vi "Test NES.vi"() -> ()   [LabVIEW 2019]
uses:
  src/Instrument.DAQ/Typedefs/Get State-enum.ctl
  src/Instrument UI.Lockin/Typedefs/UI.Configuration--Cluster.ctl
  src/Instrument.DAQ/Typedefs/Configuration.Channels--Cluster.ctl
  src/Instrument.DAQ/Typedefs/AO.Channel--Cluster--Array.ctl
  src/Instrument.DAQ/Typedefs/AO.Channel--Cluster.ctl
  src/Instrument.DAQ/Typedefs/AO.Channel.Function--Enum.ctl
  src/Instrument.DAQ/Typedefs/AI.Channel--Cluster--Array.ctl
  src/Instrument.DAQ/Typedefs/AI.Channel--Cluster.ctl
  src/Instrument.DAQ/Typedefs/REF.Channel--Cluster--Array.ctl
  src/Instrument.DAQ/Typedefs/REF.Channel--Cluster.ctl
  src/Instrument.DAQ/Typedefs/DAQ.Configuration--Cluster--Array.ctl
  src/Instrument.DAQ/Typedefs/DAQ.Configuration--Cluster.ctl
  src/Instrument.DAQ/Typedefs/DAQ.Config.AO.Range--enum.ctl
  src/Instrument.DAQ/Typedefs/DAQ.Config.AI.Range--enum.ctl
  src/Instrument.DAQ/Typedefs/DAQ.Config.AI.Coupling--enum.ctl
  src/Instrument.DAQ/Typedefs/DAQ.TerminalConfiguration--ring.ctl
  src/Instrument.DAQ/Typedefs/DAQ.Sampling--Cluster.ctl
  src/Instrument.DAQ/Typedefs/DAQ.Sampling.Sampling--Cluster.ctl
  src/Instrument.DAQ/Typedefs/DAQ.Sampling.Fs Mode--enum.ctl
  src/Instrument.DAQ/Typedefs/DAQ.Calibration--Cluster--Array.ctl
  src/Instrument.DAQ/Typedefs/DAQ.Calibration--Cluster.ctl
  src/Instrument.DAQ/Typedefs/Simulation Mode--enum.ctl
  src/Instrument.DAQ/Typedefs/Configuration.Prefilter--Cluster.ctl
  src/Instrument.DAQ/Typedefs/Channel.GainsAndOffsets--Cluster.ctl
  src/Instrument.DAQ/Typedefs/Channel.Gain--Cluster--Array.ctl
  src/Instrument.DAQ/Typedefs/Channel.Gain--Cluster.ctl
  src/Instrument.DAQ/Typedefs/Configuration.AmplitudeLimit--Cluster.ctl
  src/Instrument.DAQ/Typedefs/Configuration.DCLimit--Cluster.ctl
  src/Instrument.DAQ/Typedefs/Configuration.LinkFrequencies--Cluster.ctl
  src/Instrument.DAQ/Typedefs/Sweep.Configuration--Cluster.ctl
  src/Instrument.DAQ/Typedefs/Sweep.Channel--Cluster--Array.ctl
  src/Instrument.DAQ/Typedefs/Sweep.Channel--Cluster.ctl
  src/Instrument.DAQ/Typedefs/Sweep.Pattern--Enum.ctl
  src/Instrument UI.Lockin/Typedefs/Display-Enum.ctl
  src/Instrument.DAQ/Typedefs/Configuration.DutyCycle--Cluster.ctl
  src/Instrument UI.Lockin/Typedefs/UI.References--Cluster.ctl
  src/Instrument UI.Lockin/Typedefs/UI.References.Booleans--Cluster.ctl
  src/Instrument UI.Lockin/Typedefs/UI.References.Clusters--Cluster.ctl
  src/Instrument UI.Lockin/Typedefs/UI.References.Graphs--Cluster.ctl
  src/Instrument.Lockin/Typedefs/Lockin.getAllData--Cluster.ctl
  src/Instrument.DAQ/Typedefs/PublicEvents--DAQ.getWaveforms.ctl
  src/Instrument.DAQ/Typedefs/Results--Cluster.ctl
  src/Instrument.DAQ/Typedefs/PublicEvents--DAQ.getSweepWaveforms.ctl
  <userlib>/LevyLab/Configuration/Configuration.lvclass
  src/Instrument.DAQ/Instrument.DAQ.lvclass
  src/Instrument.Lockin/Instrument.Lockin.lvclass
  src/Instrument UI.Lockin/Instrument UI.Lockin.lvclass
  <vilib>/measure/NI_MABase.lvlib
panel:
  out "Average Time (BBN, In Place, In Place Bundle)":dbl[](array[numeric])
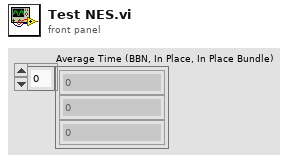
[diagram p1: front panel]
types:
  T1 = typedef "Instrument.Lockin.lvlib/Instrument.DAQ.lvclass/Get State-enum.ctl" = enum16{"idle", "created", "started", "stopped", "sweeping"}
  T2 = typedef "Instrument.Lockin.lvlib/Instrument UI.Lockin.lvclass/UI.Configuration--Cluster.ctl" = cluster{"Channels":T3, "DAQ":cluster{"Configuration":T11, "cfg.Sampling":T17, "Calibration":T20, "Simulation mode":T22}, "PreFilter":T23, "Amplifers":T24, "Limit Amplitude":T27, "Limit DC":T28, "Link Frequencies":T29, "Sweep":T30, "Plot":cluster{"visibility.AI":bool[], "visibility.AO":bool[], "visibility.Lockin":bool[], "Display 1":T34, "Display 2":T34}, "Function Option":T35}
  T3 = typedef "Instrument.Lockin.lvlib/Instrument.DAQ.lvclass/Configuration.Channels--Cluster.ctl" = cluster{"Cfg_AO":T4, "Cfg_AI":T7, "Cfg_REF":T9}
  T4 = typedef "Instrument.Lockin.lvlib/Instrument.DAQ.lvclass/AO.Channel--Cluster--Array.ctl" = T5[]
  T5 = typedef "Instrument.Lockin.lvlib/Instrument.DAQ.lvclass/AO.Channel--Cluster.ctl" = cluster{"Enable?":bool, "Channel":i32, "Amplitude":dbl, "Offset":dbl, "Frequency":dbl, "Phase":dbl, "Function":T6, "Sweeping?":bool, "Limit AC":bool, "Limit DC?":bool, "Duty Cycle":bool}
  T6 = typedef "Instrument.Lockin.lvlib/Instrument.DAQ.lvclass/AO.Channel.Function--Enum.ctl" = enum16{"sine", "square", "triangle", "saw"}
  T7 = typedef "Instrument.Lockin.lvlib/Instrument.DAQ.lvclass/AI.Channel--Cluster--Array.ctl" = T8[]
  T8 = typedef "Instrument.Lockin.lvlib/Instrument.DAQ.lvclass/AI.Channel--Cluster.ctl" = cluster{"Enable?":bool, "Channel":i32, "References":u16[], "reference index":i32}
  T9 = typedef "Instrument.Lockin.lvlib/Instrument.DAQ.lvclass/REF.Channel--Cluster--Array.ctl" = T10[]
  T10 = typedef "Instrument.Lockin.lvlib/Instrument.DAQ.lvclass/REF.Channel--Cluster.ctl" = cluster{"Enable?":bool, "Channel":i32, "Frequency":dbl, "Phase":dbl, "TC":dbl, "Roll-Off":i32}
  T11 = typedef "Instrument.Lockin.lvlib/Instrument.DAQ.lvclass/DAQ.Configuration--Cluster--Array.ctl" = T12[]
  T12 = typedef "Instrument.Lockin.lvlib/Instrument.DAQ.lvclass/DAQ.Configuration--Cluster.ctl" = cluster{"Device":string, "AO.Ch":string, "AO.Range":T13, "AI.Ch":string, "AI.Range":T14, "AI.Coupling":T15, "AI terminal config":T16, "AO terminal config":T16}
  T13 = typedef "Instrument.Lockin.lvlib/Instrument.DAQ.lvclass/DAQ.Config.AO.Range--enum.ctl" = enum16{"±0.1", "±1.0", "±10.0", ""}
  T14 = typedef "Instrument.Lockin.lvlib/Instrument.DAQ.lvclass/DAQ.Config.AI.Range--enum.ctl" = enum16{"±0.316", "±1.00", "±3.16", "±10.0", "±31.6", "±42.4", ""}
  T15 = typedef "Instrument.Lockin.lvlib/Instrument.DAQ.lvclass/DAQ.Config.AI.Coupling--enum.ctl" = u16
  T16 = typedef "Instrument.Lockin.lvlib/Instrument.DAQ.lvclass/DAQ.TerminalConfiguration--ring.ctl" = i32
  T17 = typedef "Instrument.Lockin.lvlib/Instrument.DAQ.lvclass/DAQ.Sampling--Cluster.ctl" = cluster{"Sampling":T18, "sample mode":i32, "Fs Mode":T19, "Fs Multiplier":dbl, "Refresh Rate (Hz)":dbl, "Decimation.PreDSP":i32, "Decimation.PostDSP":i32, "Fs.Output":dbl}
  T18 = typedef "Instrument.Lockin.lvlib/Instrument.DAQ.lvclass/DAQ.Sampling.Sampling--Cluster.ctl" = cluster{"Fs":dbl, "#s":i32}
  T19 = typedef "Instrument.Lockin.lvlib/Instrument.DAQ.lvclass/DAQ.Sampling.Fs Mode--enum.ctl" = enum16{"Manual", "Auto Fs", "Max Fs"}
  T20 = typedef "Instrument.Lockin.lvlib/Instrument.DAQ.lvclass/DAQ.Calibration--Cluster--Array.ctl" = T21[]
  T21 = typedef "Instrument.Lockin.lvlib/Instrument.DAQ.lvclass/DAQ.Calibration--Cluster.ctl" = cluster{"Active Device":string, "SelfCal.LastDate/Time":dbl, "SelfCal.LastTemp":dbl, "DevTemp":dbl, "calibration due?":bool}
  T22 = typedef "Instrument.Lockin.lvlib/Instrument.DAQ.lvclass/Simulation Mode--enum.ctl" = enum16{"AI = HW simulated", "AI = noise*AO", "AI = waveguide"}
  T23 = typedef "Instrument.Lockin.lvlib/Instrument.DAQ.lvclass/Configuration.Prefilter--Cluster.ctl" = cluster{"60 Hz":bool, "Low Pass":bool, "Low Pass Cutoff (Hz)":dbl}
  T24 = typedef "Instrument.Lockin.lvlib/Instrument.DAQ.lvclass/Channel.GainsAndOffsets--Cluster.ctl" = cluster{"Offset_AI":T25, "Gain_AI":T25, "Gain_AO":T25}
  T25 = typedef "Instrument.Lockin.lvlib/Instrument.DAQ.lvclass/Channel.Gain--Cluster--Array.ctl" = T26[]
  T26 = typedef "Instrument.Lockin.lvlib/Instrument.DAQ.lvclass/Channel.Gain--Cluster.ctl" = cluster{"Channel":string, "Gain":dbl}
  T27 = typedef "Instrument.Lockin.lvlib/Instrument.DAQ.lvclass/Configuration.AmplitudeLimit--Cluster.ctl" = cluster{"Limit?":bool, "Limit (V)":dbl}
  T28 = typedef "Instrument.Lockin.lvlib/Instrument.DAQ.lvclass/Configuration.DCLimit--Cluster.ctl" = cluster{"Limit?":bool, "Limit (V)":dbl}
  T29 = typedef "Instrument.Lockin.lvlib/Instrument.DAQ.lvclass/Configuration.LinkFrequencies--Cluster.ctl" = cluster{"Link?":bool, "Frequency (Hz)":dbl}
  T30 = typedef "Instrument.Lockin.lvlib/Instrument.DAQ.lvclass/Sweep.Configuration--Cluster.ctl" = cluster{"Sweep Time (s)":dbl, "Initial Wait (s)":dbl, "Return to Start":bool, "Channels":T31}
  T31 = typedef "Instrument.Lockin.lvlib/Instrument.DAQ.lvclass/Sweep.Channel--Cluster--Array.ctl" = T32[]
  T32 = typedef "Instrument.Lockin.lvlib/Instrument.DAQ.lvclass/Sweep.Channel--Cluster.ctl" = cluster{"Enable?":bool, "Channel":u16, "Start":dbl, "End":dbl, "Pattern":T33, "Table":dbl[]}
  T33 = typedef "Instrument.Lockin.lvlib/Instrument.DAQ.lvclass/Sweep.Pattern--Enum.ctl" = enum16{"Ramp /", "Ramp /\\", "Smooth Ramp _/", "Smooth Ramp _/\\_", "Table"}
  T34 = typedef "Instrument.Lockin.lvlib/Instrument UI.Lockin.lvclass/Display-Enum.ctl" = enum16{"X", "Y", "R", "Theta", "Mean"}
  T35 = typedef "Instrument.Lockin.lvlib/Instrument.DAQ.lvclass/Configuration.DutyCycle--Cluster.ctl" = cluster{"Option?":bool, "Duty Cycle (%)":dbl}
  T36 = typedef "Instrument.Lockin.lvlib/Instrument UI.Lockin.lvclass/UI.References--Cluster.ctl" = cluster{"Booleans":T37, "Clusters":T38, "Graphs":T39}
  T37 = typedef "Instrument.Lockin.lvlib/Instrument UI.Lockin.lvclass/UI.References.Booleans--Cluster.ctl" = cluster{"Start":refnum<vi>, "Pause":refnum<vi>, "Reset":refnum<vi>, "Trigger":refnum<vi>, "Help":refnum<vi>, "Close":refnum<vi>, "Start Sweep":refnum<vi>, "Stop Sweep":refnum<vi>}
  T38 = typedef "Instrument.Lockin.lvlib/Instrument UI.Lockin.lvclass/UI.References.Clusters--Cluster.ctl" = cluster{"AO Channels":refnum<vi>, "AI Channels":refnum<vi>, "REF Channels":refnum<vi>, "DAQ Config":refnum<vi>, "Sweep Channels":refnum<vi>, "Cal Info":refnum<vi>}
  T39 = typedef "Instrument.Lockin.lvlib/Instrument UI.Lockin.lvclass/UI.References.Graphs--Cluster.ctl" = cluster{"AI Graph":refnum<vi>, "AO Graph":refnum<vi>, "REF Graph":refnum<vi>, "Lockin 1":refnum<vi>, "Lockin 2":refnum<vi>, "Lockin XY":refnum<vi>, "Sweep X Graph":refnum<vi>, "Sweep Y Graph":refnum<vi>, "Sweep AI Graph":refnum<vi>, "Sweep AO Graph":refnum<vi>, "PS WFGraph":refnum<vi>, "PS Chart":refnum<vi>}
  T40 = typedef "Instrument.Lockin.lvlib/Instrument.Lockin.lvclass/Lockin.getAllData--Cluster.ctl" = cluster{"DAQ State":T1, "Waveforms":T41, "Results":T42, "SweepWaveforms":T43}
  T41 = typedef "Instrument.Lockin.lvlib/Instrument.DAQ.lvclass/PublicEvents--DAQ.getWaveforms.ctl" = cluster{"AO":waveform(dbl)[], "AI":waveform(dbl)[], "REF_X":waveform(dbl)[], "REF_Y":waveform(dbl)[], "X":waveform(dbl)[], "Y":waveform(dbl)[]}
  T42 = typedef "Instrument.Lockin.lvlib/Instrument.DAQ.lvclass/Results--Cluster.ctl" = cluster{"Time Stamp":timestamp, "Results (Dictionary)":cluster{"key":string, "value":dbl[]}[]}
  T43 = typedef "Instrument.Lockin.lvlib/Instrument.DAQ.lvclass/PublicEvents--DAQ.getSweepWaveforms.ctl" = cluster{"AO":waveform(dbl)[], "AI":waveform(dbl)[], "X":waveform(dbl)[], "Y":waveform(dbl)[]}
  T44 = cluster{"Configuration":refnum<class "Configuration.lvclass">, "UI Config":T2, "DAQ state":T1, "getAll":T40, "References":T36, "Message":cluster{"Command":variant, "Data":variant}, "Plot Names":string[], "Front Panel":refnum<vi>, "update graphs":bool}
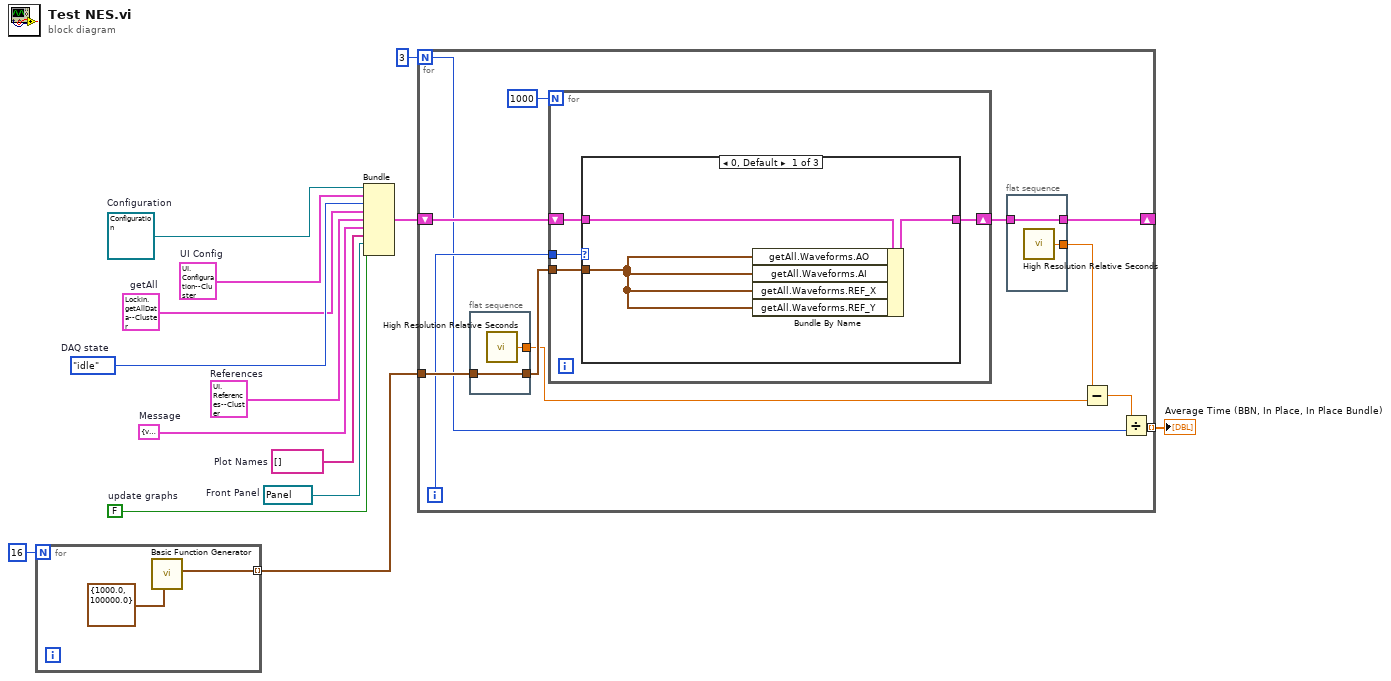
[diagram p0: block diagram]
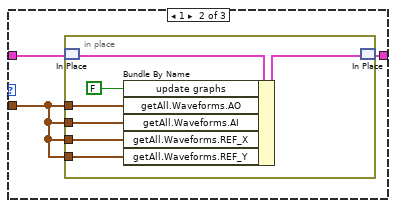
[diagram p2: hidden frame]
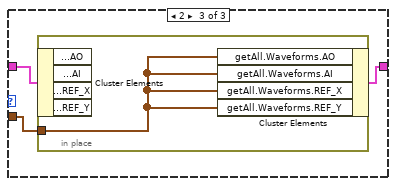
[diagram p3: hidden frame]
diagram:
  w6 = FALSE  # update graphs
  w8 = Get_State-enum."idle"  # DAQ state
  w9 = refnum<vi> refnum  # Front Panel
  w11 = T2 {"Channels"={"Cfg_AO"=[], "Cfg_AI"=[], "Cfg_REF"=[]}, "DAQ"={"Configuration"=[], "cfg.Sampling"={"Sampling"={"Fs"=0.0, "#s"=0}, "sample mode"=0, "Fs Mode"=enum."Manual", "Fs Multiplier"=0.0, "Refresh Rate (Hz)"=0.0, "Decimation.PreDSP"=0, "Decimation.PostDSP"=0, "Fs.Output"=204789.0}, "Calibration"=[], "Simulation mode"=enum."AI = HW simulated"}, "PreFilter"={"60 Hz"=FALSE, "Low Pass"=FALSE, "Low Pass Cutoff (Hz)"=0.0}, "Amplifers"={"Offset_AI"=[], "Gain_AI"=[], "Gain_AO"=[]}, "Limit Amplitude"={"Limit?"=FALSE, "Limit (V)"=0.0}, "Limit DC"={"Limit?"=FALSE, "Limit (V)"=0.0}, "Link Frequencies"={"Link?"=FALSE, "Frequency (Hz)"=0.0}, "Sweep"={"Sweep Time (s)"=0.0, "Initial Wait (s)"=0.0, "Return to Start"=FALSE, "Channels"=[]}, "Plot"={"visibility.AI"=[], "visibility.AO"=[], "visibility.Lockin"=[], "Display 1"=enum."X", "Display 2"=enum."X"}, "Function Option"={"Option?"=FALSE, "Duty Cycle (%)"=0.0}}  # UI Config
  w10 = string[] []  # Plot Names
  w14 = T36 {"Booleans"={"Start"=refnum, "Pause"=refnum, "Reset"=refnum, "Trigger"=refnum, "Help"=refnum, "Close"=refnum, "Start Sweep"=refnum, "Stop Sweep"=refnum}, "Clusters"={"AO Channels"=refnum, "AI Channels"=refnum, "REF Channels"=refnum, "DAQ Config"=refnum, "Sweep Channels"=refnum, "Cal Info"=refnum}, "Graphs"={"AI Graph"=refnum, "AO Graph"=refnum, "REF Graph"=refnum, "Lockin 1"=refnum, "Lockin 2"=refnum, "Lockin XY"=refnum, "Sweep X Graph"=refnum, "Sweep Y Graph"=refnum, "Sweep AI Graph"=refnum, "Sweep AO Graph"=refnum, "PS WFGraph"=refnum, "PS Chart"=refnum}}  # References
  w12 = cluster{"Command":variant, "Data":variant} {"Command"=variant, "Data"=variant}  # Message
  w7 = T40 {"DAQ State"=enum."idle", "Waveforms"={"AO"=[], "AI"=[], "REF_X"=[], "REF_Y"=[], "X"=[], "Y"=[]}, "Results"={"Time Stamp"=timestamp(0 s since 1904-01-01), "Results (Dictionary)"=[]}, "SweepWaveforms"={"AO"=[], "AI"=[], "X"=[], "Y"=[]}}  # getAll
  w13 = refnum<class "Configuration.lvclass"> refnum  # Configuration
  n1 = for {
    N: 16 -> [_]
    tunnel: [w15] -> w3 mode=indexing
    n2 = call <vilib>:"Basic Function Generator.vi"("sampling info"=cluster{"Fs":dbl, "#s":dbl} {"Fs"=1000.0, "#s"=100000.0}) -> ("signal out"=w15:waveform(dbl))  [unwired: 8 in, 2 out]
  }
  n3 = Bundle("Configuration"=w13, "UI Config"=w11, "DAQ state"=w8, "getAll"=w7, "References"=w14, "Message"=w12, "Plot Names"=w10, "Front Panel"=w9, "update graphs"=w6) -> (w5:T44)  [unwired: 1 in]
  n4 = for {
    N: 3 -> [w18]
    tunnel: w3 -> [w25]
    shift-right: [w23] -> _
    shift-left: w5 -> [w28]
    tunnel: [w17] -> w1 mode=indexing
    i -> [w22]
    n5 = flat-sequence {
      tunnel: w25 -> [w32]
      tunnel: [w32] -> w26
      tunnel: [w31] -> w20
      frame #0 {
        n6 = call <vilib>:"High Resolution Relative Seconds.vi"() -> ("relative seconds"=w31:dbl)
      }
    }
    n7 = for {
      N: 1000 -> [_]
      tunnel: w26 -> [w35]
      shift-right: [w34] -> w24
      shift-left: w28 -> [w36]
      tunnel: w22 -> [w33]
      n8 = case shown="0, Default" w33 {
        tunnel: w36 -> [w39 w42 w52]
        tunnel: w35 -> [w37 w41 w50]
        tunnel: [w38 w40 w51] -> w34
        frame 0, Default {
          n9 = Bundle By Name(cluster=w39, "getAll.Waveforms.AO"=w37, "getAll.Waveforms.AI"=w37, "getAll.Waveforms.REF_X"=w37, "getAll.Waveforms.REF_Y"=w37) -> (w38:T44)
        }
        frame 1 {
          n10 = in-place {
            in-place-border: w41 -> [w49]
            in-place-border: w41 -> [w48]
            in-place-border: w41 -> [w47]
            in-place-border: w41 -> [w46]
            n11 = in-place-match #1(w42) -> (w44:T44)
            n12 = Bundle By Name(cluster=w44, "update graphs"=FALSE, "getAll.Waveforms.AO"=w46, "getAll.Waveforms.AI"=w49, "getAll.Waveforms.REF_X"=w48, "getAll.Waveforms.REF_Y"=w47) -> (w43:T44)
            n13 = in-place-match #1(w43) -> (w40:T44)
          }
        }
        frame 2 {
          n14 = in-place {
            in-place-border: w50 -> [w53]
            n15 = in-place-cluster #2(w52) -> ()  [unwired: 4 out]
            n16 = in-place-cluster #2("getAll.Waveforms.AO"=w53, "getAll.Waveforms.AI"=w53, "getAll.Waveforms.REF_X"=w53, "getAll.Waveforms.REF_Y"=w53) -> (w51:T44)
          }
        }
      }
    }
    n17 = flat-sequence {
      tunnel: w24 -> [w30]
      tunnel: [w30] -> w23
      tunnel: [w29] -> w21
      frame #0 {
        n18 = call <vilib>:"High Resolution Relative Seconds.vi"() -> ("relative seconds"=w29:dbl)
      }
    }
    n19 = Subtract(x=w21, y=w20) -> (x-y=w19:dbl)
    n20 = Divide(x=w19, y=w18) -> (x/y=w17:dbl)
  }
  "Average Time (BBN, In Place, In Place Bundle)" <- w1
